vi "Update Configure NF Steps.vi"(7 "Steps to Update":string[](array[string]), 8 "error in (no error)":errorcluster, 9 "Configure NF Sequence Ref":refnum<k7>, 11 "NF in":refnum<class "NF.lvclass">) -> (0 "error out":errorcluster, 1 "Configure NF Sequence Ref":refnum<k7>, 3 "NF out":refnum<class "NF.lvclass">)   [LabVIEW 2018, in "NF.lvlib" / "NF.lvclass"]
uses:
  NF.lvclass
  Plugins/Measurement Interface.lvlibp/Measurement Interface.lvclass
  Plugins/TestStand API Tools (TSAT).lvlibp/Sequence Actions/TSAT Sequence Actions.lvlib
  C:/Sequence Automation/Plugins/Measurement Interface.lvlibp/Measurement Interface.lvclass
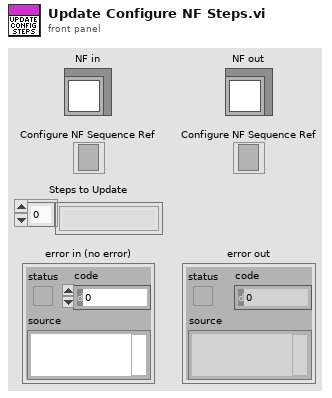
[diagram p1: front panel]
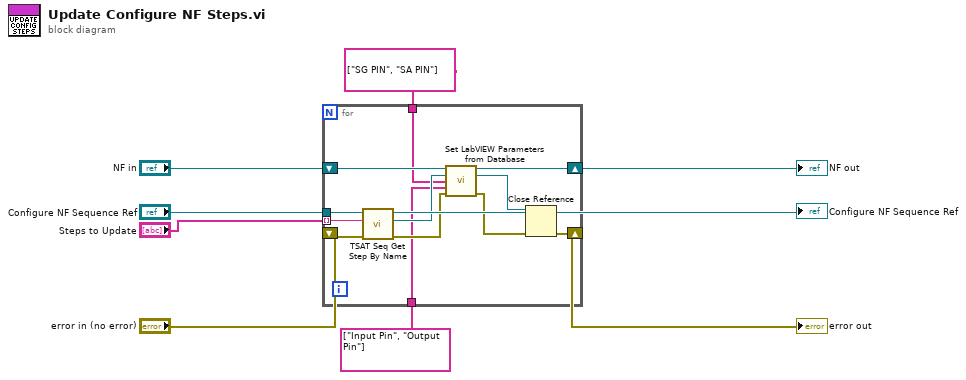
[diagram p0: block diagram]
diagram:
  n1 = for {
    tunnel: "Configure NF Sequence Ref" -> [w20]
    tunnel: "Steps to Update" -> [w17] mode=indexing
    shift-right: [w16] -> w4
    shift-left: "NF in" -> [w15]
    tunnel: string[] ["SG PIN", "SA PIN"] ("Dictionary Keys") -> [w11]
    tunnel: string[] ["Input Pin", "Output Pin"] ("LabVIEW Parameter Mapping") -> [w10]
    shift-right: [w9] -> w1
    shift-left: "error in (no error)" -> [w18]
    n2 = call "TSAT Seq Get Step By Name.vi"("Error In"=w18, "Step name"=w17, "Sequence Reference In"=w20) -> ("Error Out"=w12:errorcluster, "Step Reference Out"=w19:refnum<k7>)  [unwired: 6 in, 1 out]
    n3 = call "Set LabVIEW Parameters from Database.vi"("Measurement Interface in"=w15, "Step In"=w19, "Dictionary Keys"=w11, "LabVIEW Parameter Mapping"=w10, "error in (no error)"=w12) -> ("Measurement Interface out"=w16:refnum<class "NF.lvclass">, "Step Out"=w14:refnum<k7>, "error out"=w13:errorcluster)  [unwired: 8 in]
    n4 = Close Reference(reference=w14, error in (no error)=w13) -> (error out=w9:errorcluster)
  }
  "error out" <- w1
  "NF out" <- w4
  "Configure NF Sequence Ref" <- "Configure NF Sequence Ref"
